vi "New Logger.vi"(7 "Logger Name":string, 8 "error in (no error)":errorcluster, 11 "Logger Output in":T1) -> (0 "error out":errorcluster)   [LabVIEW 2016, in "Global_logger.lvlib"]
uses:
  Global_logger.lvlib
  Logger Output.ctl
  Levels.ctl
  Level Meaning.ctl
  Sorting.ctl
  Logger Type.ctl
  Log Fields.ctl
  Event.ctl
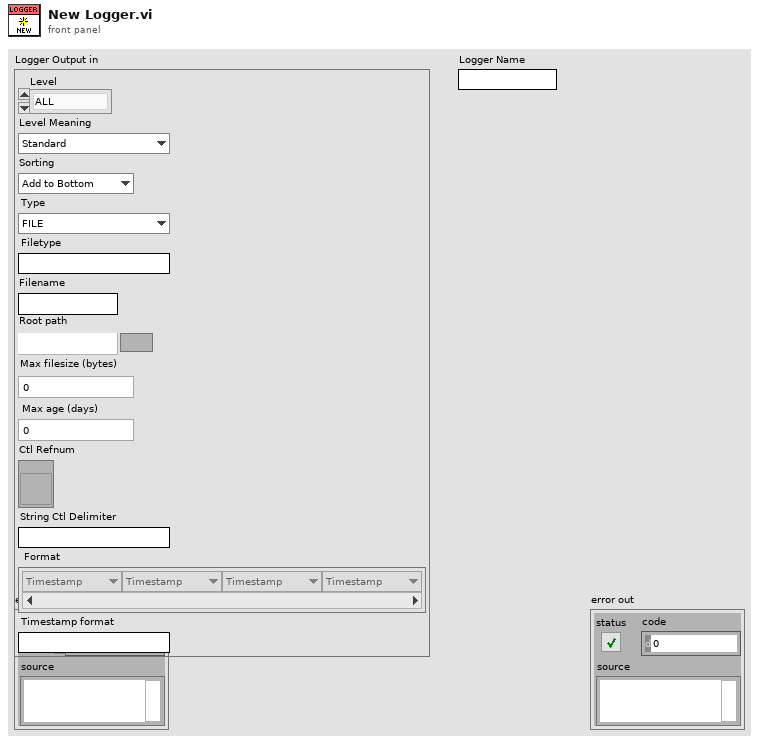
[diagram p1: front panel]
types:
  T1 = typedef "Global_logger.lvlib/Logger Output.ctl" = cluster{"Level":T2, "Level Meaning":T3, "Sorting":T4, "Type":T5, "Filetype":string, "Filename":string, "Root path":path, "Max filesize (bytes)":i32, "Max age (days)":i32, "Ctl Refnum":refnum<vi>, "String Ctl Delimiter":string, "Format":T6[], "Timestamp format":string}
  T2 = typedef "Global_logger.lvlib/Levels.ctl" = enum16{"ALL", "TRACE", "DEBUG", "INFO", "WARN", "ERROR", "FATAL", "OFF"}
  T3 = typedef "Global_logger.lvlib/Level Meaning.ctl" = enum16{"Standard", "Positive", "Exact"}
  T4 = typedef "Global_logger.lvlib/Sorting.ctl" = enum16{"Add to Bottom", "Add to Top"}
  T5 = typedef "Global_logger.lvlib/Logger Type.ctl" = enum16{"FILE", "UI"}
  T6 = typedef "Global_logger.lvlib/Log Fields.ctl" = enum16{"Timestamp", "Level", "Message", "Source VI", "Source App", "Logger Name"}
  T7 = typedef "Global_logger.lvlib/Event.ctl" = cluster{"Logger Name":string, "Time Stamp":timestamp, "Level":T2, "Source VI":string, "Message":string, "Source App":string}
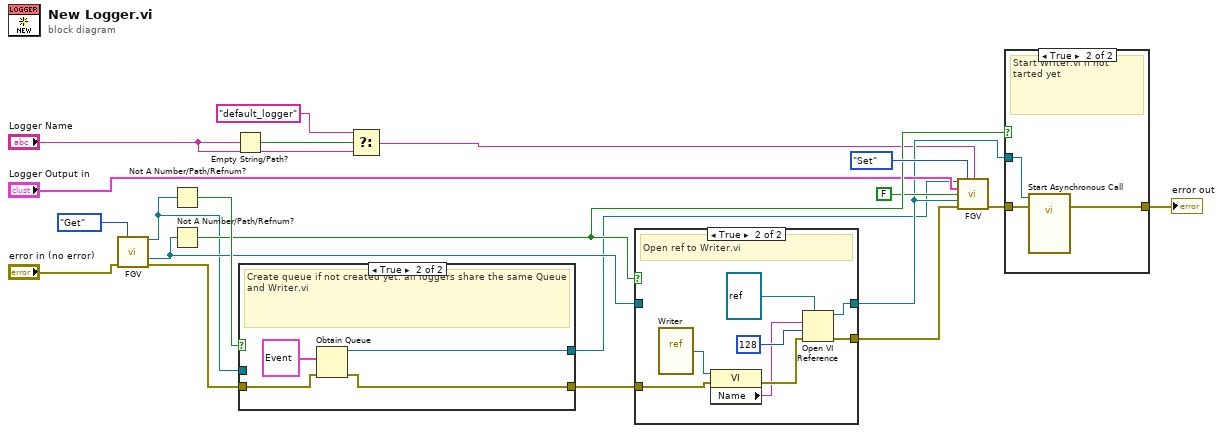
[diagram p0: block diagram]
diagram:
  n1 = call "FGV.vi"("Action"=enum16{"Get", "Set"}."Get", "error in (no error)"="error in (no error)") -> ("queue out"=w6:refnum<queue>, "Writer ref out"=w14:refnum<vi>, "error out"=w11:errorcluster)  [unwired: 8 in, 3 out]
  n2 = Not A Number/Path/Refnum?(number/path/refnum=w6) -> (NaN/Path/Refnum?=w15:bool)
  n3 = Not A Number/Path/Refnum?(number/path/refnum=w14) -> (NaN/Path/Refnum?=w13:bool)
  n4 = Empty String/Path?(string/path="Logger Name") -> (empty?=w4:bool)
  n5 = case shown="True" w15 {
    tunnel: [w22 w23] -> w5
    tunnel: w6 -> [w22 _]
    tunnel: w11 -> [w21 w25]
    tunnel: [w21 w24] -> w10
    frame False {
    }
    frame True {
      # "Create queue if not created yet: all loggers share the same Queue and Writer.vi"
      n6 = Obtain Queue(element data type=T7 {"Logger Name"="", "Time Stamp"=timestamp(0 s since 1904-01-01), "Level"=enum."ALL", "Source VI"="", "Message"="", "Source App"=""} ("Event"), error in (no error)=w25) -> (queue out=w23:refnum<queue>, error out=w24:errorcluster)  [unwired: 3 in, 1 out]
    }
  }
  n7 = Select(t="default_logger", s=w4, f="Logger Name") -> (s? t:f=w3:string)
  n8 = case shown="True" w13 {
    tunnel: [w28 w31] -> w7
    tunnel: w14 -> [w28 _]
    tunnel: [w27 w30] -> w12
    tunnel: w10 -> [w27 w29]
    frame False {
    }
    frame True {
      # "Open ref to Writer.vi"
      n9 = vi-ref "Writer.vi"() -> (w32:refnum<vi>)
      n10 = property class="VI"(reference=w32, error in=w29) -> (error out=w35:errorcluster, "Name"=w33:string)  [unwired: 1 out]
      n11 = Open VI Reference(type specifier VI Refnum (for type only)=refnum<vi> refnum, vi path=w33, options=128, error in (no error)=w35) -> (vi reference=w31:refnum<vi>, error out=w30:errorcluster)  [unwired: 2 in]
    }
  }
  n12 = call "FGV.vi"("queue in"=w5, "Action"=enum16{"Get", "Set"}."Set", "Logger Name"=w3, "Logger Output in"="Logger Output in", "Destroy Logger in"=FALSE, "Writer ref in"=w7, "error in (no error)"=w12) -> ("error out"=w18:errorcluster)  [unwired: 3 in, 5 out]
  n13 = case shown="True" w13 {
    tunnel: [w37 w40] -> w20
    tunnel: w18 -> [w37 w39]
    tunnel: w7 -> [_ w38]
    frame False {
    }
    frame True {
      # "Start Writer.vi if not tarted yet"
      n14 = call-by-ref "Start Asynchronous Call"(reference=w38, error in=w39) -> (error out=w40:errorcluster)  [unwired: 12 in, 1 out]
    }
  }
  "error out" <- w20
